vi "MARS_Plot_Scan_Ratio.vi"(9 "Total Integral":i32[](array[numeric]), 10 "Tail Integral in":i32[](array[numeric]), 11 "IntensityGraph in":refnum<vi>) -> (2 "Histogram":i32[](array[numeric]), 3 "Ratio Graph":i32[][](graph))   [LabVIEW 2015]
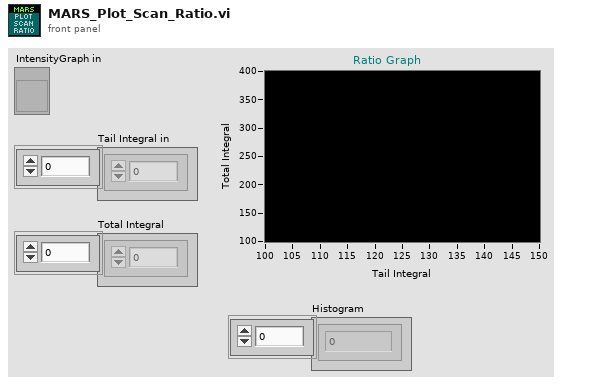
[diagram p1: front panel]
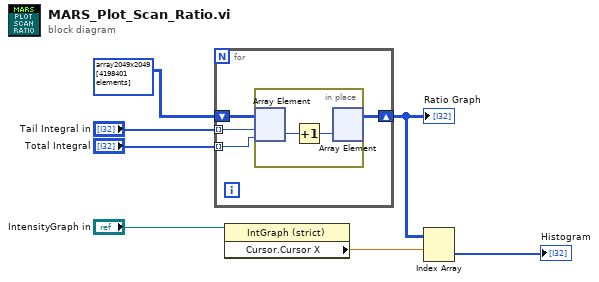
[diagram p0: block diagram]
diagram:
  n1 = for {
    tunnel: "Tail Integral in" -> [w10] mode=indexing
    shift-right: [w8] -> w6
    shift-left: i32[][] array2049x2049[4198401 elements] ("Tail Integral") -> [w11]
    tunnel: "Total Integral" -> [w9] mode=indexing
    n2 = in-place {
      n3 = in-place-array #1(w11, w10, w9) -> (w13:i32)
      n4 = Increment(x=w13) -> (x+1=w12:i32)
      n5 = in-place-array #1(w12) -> (w8:i32[][])  [unwired: 2 out]
    }
  }
  "Ratio Graph" <- w6
  n6 = property on="Property Node" class="IntGraph (strict)"(reference="IntensityGraph in") -> ("Cursor.Cursor X"=w4:dbl)  [unwired: 1 in, 2 out]
  n7 = Index Array(array=w6, index (row)=w4) -> (element=→"Histogram":i32[])  [unwired: 1 in]
